vi "Close Wrist.vi"(8 "error in (no error)":errorcluster) -> (0 "error out":errorcluster)   [LabVIEW 2018]
uses:
  TypeDefs/typedef_enum_Refnums.ctl
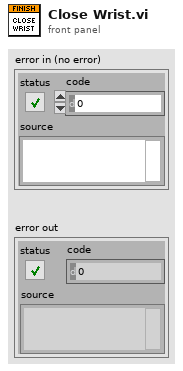
[diagram p1: front panel]
types:
  T1 = typedef "typedef_enum_Refnums.ctl" = enum16{"Ball_Encoder", "Ball_Motor", "Camera", "Linefollow_3", "Linefollow_2", "Linefollow_1", "Gyro", "Hatch_Solenoid", "Climb_Back_Solenoid", "Arm_Encoder", "Arm_Motor", "Lift_Encoder", "Arm_Motor_R", "Arm_Motor_L", "Drive", "Drive_Motor_R", "Drive_Motor_L", "Drive_Encoder_R", "Drive_Encoder_L", "Joy_R", "Joy_L", "Wrist_Motor", "Wrist_Encoder", "Climb_Front_Encoder", "Climb_Front_Motor"}
  T2 = typedef "WPI_MotorControlDeviceRef.ctl" = cluster{"DeviceStatus":errorcluster, "Type":T3, "PWM":cluster{"PWM Channel":T4, "DeadBand":T5}, "CAN":cluster{"Device Number":u8, "SetOutput VI Ref":variant, "GetOutput VI Ref":variant, "Enable VI Ref":variant, "Disable VI Ref":variant, "Data":variant}, "Invert":bool, "DIO PWM":cluster{"PWM \"Enable\" Channel":T4, "DIOChannel":T6, "PWM Rate":dbl}}
  T3 = typedef "WPI_MotorControlType.ctl" = enum16{"PWM", "CAN", "DIO PWM"}
  T4 = typedef "FPGA_DIOPWMChannel.ctl" = enum8{"PWM 0", "PWM 1", "PWM 2", "PWM 3", "PWM 4", "PWM 5", "PWM 6", "PWM 7", "PWM 8", "PWM 9", "PWM MXP 0", "PWM MXP 1", "PWM MXP 2", "PWM MXP 3", "PWM MXP 4", "PWM MXP 5", "PWM MXP 6", "PWM MXP 7", "PWM MXP 8", "PWM MXP 9", "Invalid"}
  T5 = typedef "WPI_PWMDeadband.ctl" = cluster{"Name":string, "maxPositivePwm":i32, "minPositivePwm":i32, "centerPwm":i32, "maxNegativePwm":i32, "minNegativePwm":i32, "angularRange":u16}
  T6 = typedef "FPGA_DIOChannel.ctl" = enum8{"DIO 0", "DIO 1", "DIO 2", "DIO 3", "DIO 4", "DIO 5", "DIO 6", "DIO 7", "DIO 8", "DIO 9", "DIO MXP 0", "DIO MXP 1", "DIO MXP 2", "DIO MXP 3", "DIO MXP 4", "DIO MXP 5", "DIO MXP 6", "DIO MXP 7", "DIO MXP 8", "DIO MXP 9", "DIO MXP 10", "DIO MXP 11", "DIO MXP 12", "DIO MXP 13", "DIO MXP 14", "DIO MXP 15", "SPI Port CS1", "SPI Port CS2", "SPI Port CS3", "SPI Port MISO", "SPI Port MOSI", "Invalid"}
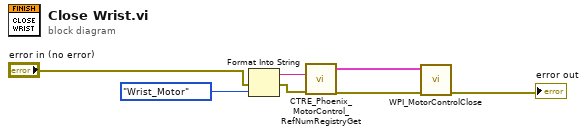
[diagram p0: block diagram]
diagram:
  n1 = Format Into String(error in="error in (no error)", typedef_enum_Refnums."Wrist_Motor" ("RefNums")) -> (resulting string=w6:string, error out=w7:errorcluster)  [unwired: 2 in]
  n2 = call <vilib>:"CTRE_Phoenix_MotorControl_RefNumRegistryGet.vi"("error in (no error)"=w7, "refnum name"=w6) -> ("error out"=w2:errorcluster, "PhoenixMotorControlDevRef"=w3:T2)  [unwired: 8 in]
  n3 = call <vilib>:"WPI_MotorControlClose.vi"("error in"=w2, "MotorControlDevRef"=w3) -> ("error out"=→"error out":errorcluster)  [unwired: 9 in]
